vi "Areotech set speed.vi"(8 "error in (no error)":errorcluster, 10 "Parsed CMD":T1, 11 "AerotechStage in":refnum<class "AerotechStage.lvclass">) -> (0 "error out":errorcluster, 2 "new commands":string, 3 "AerotechStage out":refnum<class "AerotechStage.lvclass">)   [LabVIEW 2020, in "AerotechStage.lvclass"]
uses:
  AerotechStage.lvclass
  shared/parsed device cmd.ctl
  AerotechStage.lvclass/AerotechStage.ctl
  shared/CompressAndUpdate(Poly)/CompressAndUpdate(Numeric).vi
  Sample Vis/Parameters/SetAxisParameterDouble.vi
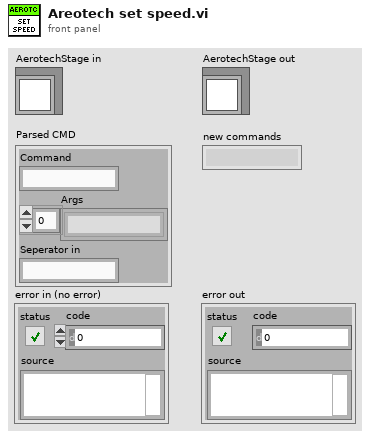
[diagram p1: front panel]
types:
  T1 = typedef "parsed device cmd.ctl" = cluster{"Command":string, "Args":string[], "Seperator in":string}
  T2 = typedef "OnOffTypeDef.ctl" = enum16{"off", "on"}
  T3 = cluster{"Axis1":cluster{"Value":dbl, "Min":dbl, "Max":dbl, "StepSize":dbl, "Tolerance":dbl, "ValueActual":dbl}, "Axis2":cluster{"Value":dbl, "Min":dbl, "Max":dbl, "StepSize":dbl, "Tolerance":dbl, "ValueActual":dbl}, "Axis3":cluster{"Value":dbl, "Min":dbl, "Max":dbl, "StepSize":dbl, "Tolerance":dbl, "ValueActual":dbl}}
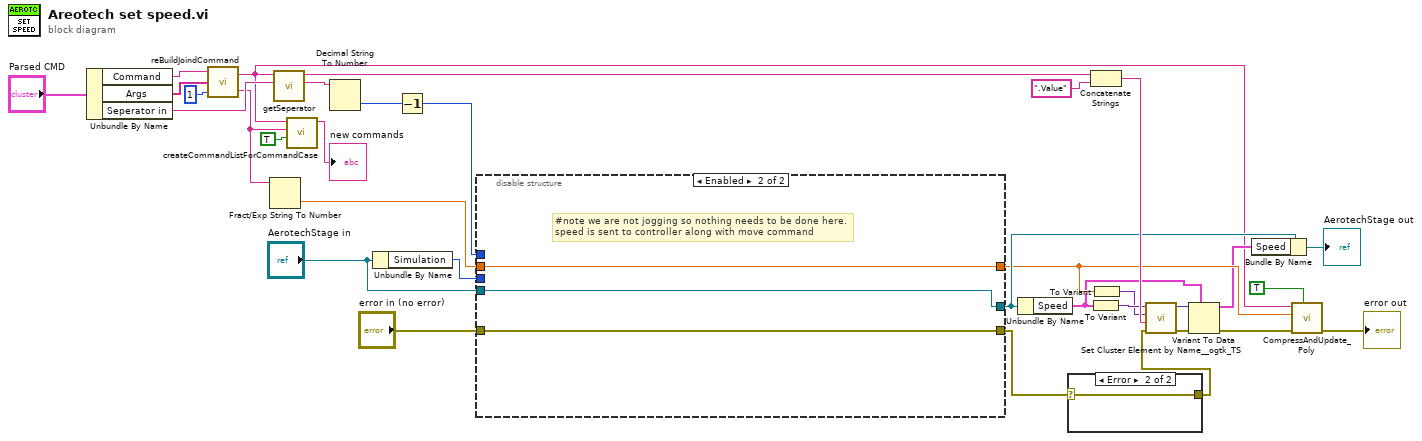
[diagram p0: block diagram]
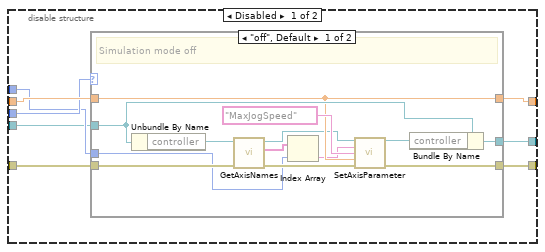
[diagram p3: hidden frame]
diagram:
  n1 = Unbundle By Name("Parsed CMD") -> ("Command"=w31:string, "Args"=w32:string[], "Seperator in"=w33:string)
  n2 = call "reBuildJoindCommand.vi"("number of group elements (0)"=1, "Args"=w32, "Command 2"=w31) -> ("Arg"=w8:string, "Command"=w6:string)
  n3 = Fract/Exp String To Number(string=w8) -> (number=w9:dbl)  [unwired: 3 in, 1 out]
  n4 = call "getSeperator.vi"("Channel Seperator (\"\")"=w33, "Command"=w6) -> ("Channel"=w13:string, "Seperator (e.g. \"Channel1\")"=w26:string)  [unwired: 8 in]
  n5 = call "createCommandListForCommandCase.vi"("immediate Check (only once)"=TRUE, "setvalue"=w8, "command"=w6) -> ("new commands"=→"new commands":string)  [unwired: 8 in]
  n6 = Decimal String To Number(string=w13) -> (number=w11:i32)  [unwired: 2 in, 1 out]
  n7 = Unbundle By Name("AerotechStage in") -> ("Simulation"=w10:T2)
  n8 = Decrement(x=w11) -> (x-1=w12:i32)
  n9 = disable-structure shown="Enabled" {
    disable-tunnel: w9 -> [w41 w59]
    disable-tunnel: w10 -> [w40 _]
    disable-tunnel: w12 -> [w39 _]
    disable-tunnel: "error in (no error)" -> [w38 w60]
    disable-tunnel: [w37 w59] -> w21
    disable-tunnel: "AerotechStage in" -> [w36 w58]
    disable-tunnel: [w35 w58] -> w23
    disable-tunnel: [w34 w60] -> w1
    frame Disabled {
      n10 = case shown="\"off\", Default" w40 {
        tunnel: w41 -> [w49 w56]
        tunnel: w36 -> [w52 w57]
        tunnel: [w53 w55] -> w34
        tunnel: [w50 w57] -> w35
        tunnel: [w49 w56] -> w37
        tunnel: w38 -> [w46 w55]
        tunnel: w39 -> [w44 _]
        frame "off", Default {
          # "Simulation mode off"
          n11 = Unbundle By Name(w52) -> ("controller"=w48:refnum<k24>)
          n12 = call "GetAxisNames.vi"("error in (no error)"=w46, "controller in"=w48) -> ("error out"=w47:errorcluster, "axis names"=w45:string[], "controller out"=w42:refnum<k24>)  [unwired: 7 in]
          n13 = Index Array(array=w45, index=w44) -> (element=w43:string)
          n14 = call-poly "SetAxisParameter.vi"("Controller In"=w42, "axisName"=w43, "Parameter Name"="MaxJogSpeed", "value"=w49, "error in (no error)"=w47) -> ("Controller Out"=w51:refnum<k24>, "error out"=w53:errorcluster)  [unwired: 9 in]
          n15 = Bundle By Name(cluster=w52, "controller"=w51) -> (w50:refnum<class "AerotechStage.lvclass">)
        }
        frame "on" {
          # "Simulation mode on"
        }
      }
    }
    frame Enabled {
      # "#note we are not jogging so nothing needs to be done here.\nspeed is sent to controller along with move command"
    }
  }
  n16 = Unbundle By Name(w23) -> ("Speed"=w16:T3)
  n17 = case shown="Error" w1 {
    selector: w1 -> [_ w61]
    tunnel: [_ w61] -> w2
    frame No Error {
    }
    frame Error {
    }
  }
  n18 = Concatenate Strings(w26, ".Value" ("string")) -> (w27:string)
  n19 = To Variant(anything=w16) -> (Variant=w19:variant)
  n20 = To Variant(anything=w21) -> (Variant=w18:variant)
  n21 = call "Set Cluster Element by Name__ogtk_TS.vi"("error in (no error)"=w2, "Element Name (\"\": New Element Data Name)"=w27, "New Element Value"=w18, "Cluster"=w19) -> ("error out"=w14:errorcluster, "VCluster out"=w15:variant)  [unwired: 5 in, 1 out]
  n22 = Variant To Data(error in=w14, type=w16, Variant=w15) -> (data=w17:T3, error out=w29:errorcluster)
  n23 = Bundle By Name(cluster=w23, "Speed"=w17) -> (→"AerotechStage out":refnum<class "AerotechStage.lvclass">)
  n24 = call-poly "CompressAndUpdate_Poly.vi"("force CVT update (false)"=TRUE, "error in"=w29, "Numeric"=w21, "command or variable name"=w6) -> ("error out"=→"error out":errorcluster)  [unwired: 7 in]
